vi "Time_for_measure.vi"(10 "Rozliseni 34401A":T1(ring), 11 "Rozliseni 34450":enum16{"4_1/2 fast", "4_1/2 slow", "5_1/2 fast"}(ring)) -> (3 "Time for measure":u32)   [LabVIEW 2021]
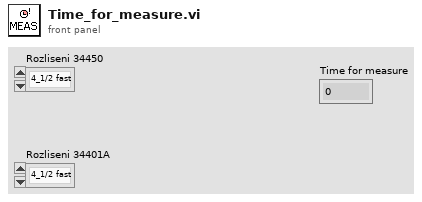
[diagram p1: front panel]
types:
  T1 = enum16{"4_1/2 fast", "4_1/2 slow", "5_1/2 fast", "5_1/2 slow", "6_1/2 fast", "6_1/2 slow"}
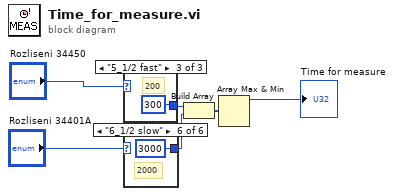
[diagram p0: block diagram]
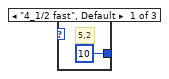
[diagram p2: hidden frame]
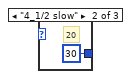
[diagram p3: hidden frame]
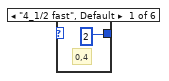
[diagram p4: hidden frame]
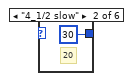
[diagram p5: hidden frame]
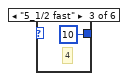
[diagram p6: hidden frame]
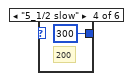
[diagram p7: hidden frame]
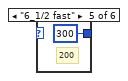
[diagram p8: hidden frame]
diagram:
  n1 = case shown="\"5_1/2 fast\"" "Rozliseni 34450" {
    tunnel: [u32 10 ("milliseconds to wait") u32 30 ("milliseconds to wait") u32 300 ("milliseconds to wait")] -> w4
    frame "4_1/2 fast", Default {
      # "5,2"
    }
    frame "4_1/2 slow" {
      # "20"
    }
    frame "5_1/2 fast" {
      # "200"
    }
  }
  n2 = case shown="\"6_1/2 slow\"" "Rozliseni 34401A" {
    tunnel: [u32 2 ("milliseconds to wait") u32 30 ("milliseconds to wait") u32 10 ("milliseconds to wait") u32 300 ("milliseconds to wait") u32 300 ("milliseconds to wait") u32 3000 ("milliseconds to wait")] -> w3
    frame "4_1/2 fast", Default {
      # "0,4"
    }
    frame "4_1/2 slow" {
      # "20"
    }
    frame "5_1/2 fast" {
      # "4"
    }
    frame "5_1/2 slow" {
      # "200"
    }
    frame "6_1/2 fast" {
      # "200"
    }
    frame "6_1/2 slow" {
      # "2000"
    }
  }
  n3 = Build Array(w4, w3) -> (w5:u32[])
  n4 = Array Max & Min(array=w5) -> (max value=→"Time for measure":u32)  [unwired: 3 out]
